vi "Files_names_v02.vi"(2 "actualSamples\narray":i32[](array[numeric]), 3 "Type of\nmeasurement":T1, 4 "Name root":string, 5 "File location":path) -> (0 "Files path array":path[](array[path]), 1 "Files name array":string[](array[string]))   [LabVIEW 2013]
uses:
  Strict Type Defs/type_meas_enum.ctl
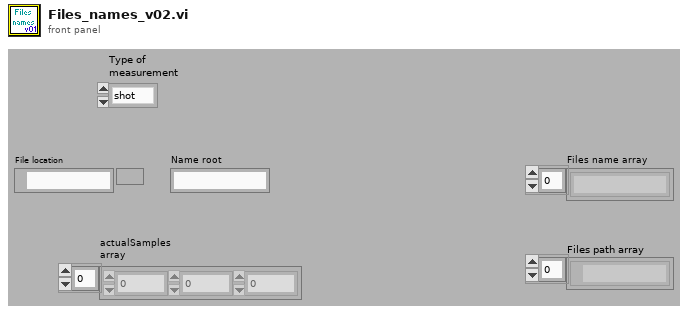
[diagram p1: front panel]
types:
  T1 = typedef "type_meas_enum.ctl" = enum16{"shot", "x", "p", "electronic"}
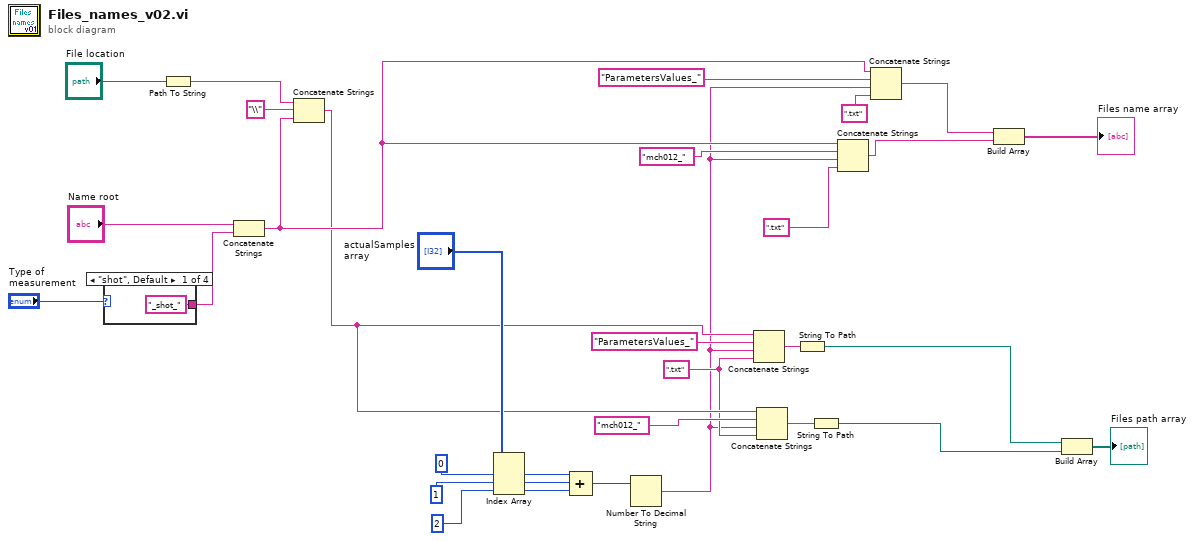
[diagram p0: block diagram]
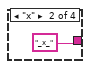
[diagram p2: hidden frame]
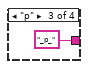
[diagram p3: hidden frame]
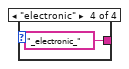
[diagram p4: hidden frame]
diagram:
  w3 = ".txt" ("string")
  n1 = case shown="\"shot\", Default" "Type of\nmeasurement" {
    tunnel: ["_shot_" "_x_" "_p_" "_electronic_"] -> w26
    frame "shot", Default {
    }
    frame "x" {
    }
    frame "p" {
    }
    frame "electronic" {
    }
  }
  n2 = Path To String(path="File location") -> (string=w21:string)
  n3 = Concatenate Strings("Name root", w26) -> (w12:string)
  n4 = Concatenate Strings(w21, "\\" ("string"), w12) -> (w11:string)
  n5 = Index Array(array="actualSamples\narray", index #1=0 ("index"), index #2=1 ("index"), index #3=2 ("index")) -> (element #1=w8:i32, element #2=w7:i32, element #3=w6:i32)
  n6 = Compound Arithmetic op=ADD(w8, w7, w6) -> (w5:i32)
  n7 = Number To Decimal String(number=w5) -> (decimal integer string=w2:string)  [unwired: 1 in]
  n8 = Concatenate Strings(w11, "ParametersValues_" ("string"), w2, w3) -> (w31:string)
  n9 = Concatenate Strings(w11, "mch012_" ("string"), w2, w3) -> (w15:string)
  n10 = String To Path(string=w31) -> (path=w18:path)
  n11 = String To Path(string=w15) -> (path=w4:path)
  n12 = Concatenate Strings(w12, "mch012_" ("string"), w2, ".txt") -> (w1:string)
  n13 = Concatenate Strings(w12, "ParametersValues_" ("string"), w2, ".txt" ("string")) -> (w20:string)
  n14 = Build Array(w20, w1) -> (→"Files name array":string[])
  n15 = Build Array(w18, w4) -> (→"Files path array":path[])
